vi "Page_Source_Can_Add_to_Top.vi"(6 "Project Refnum":refnum<vi>, 8 "error in (no error)":errorcluster, 10 "AB_Source in":refnum<class "AB_Source.lvclass">, 11 "AB_SourceDistribution in":refnum<class "AB_SourceDistribution.lvclass">) -> (0 "error out":errorcluster, 1 "message":string, 2 "canAddToTop":bool, 3 "AB_SourceDistribution out":refnum<class "AB_SourceDistribution.lvclass">)   [LabVIEW 2020, in "AB_SourceDistribution.lvclass"]
uses:
  <vilib>/AppBuilder/AB_Classes/SourceDistribution/AB_SourceDistribution.lvclass
  <vilib>/AppBuilder/AB_Classes/Source/AB_Source.lvclass
  <resource>/Framework/Providers/Common/provcom_StringGlobals.vi
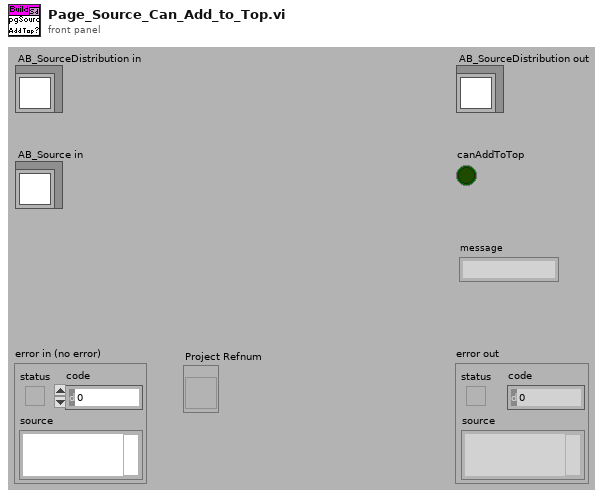
[diagram p1: front panel]
types:
  T1 = typedef "AB_Source.ctl" = cluster{"path":path, "itemID":string, "parentIndex":i32, "sourceInclusion":T2, "destinationIndex":i32, "properties":T3[], "newName":string, "lvfile":bool, "valid":bool, "eng_inBuild":bool, "eng_isNonVILink":bool, "Amalgamation":bool, "Amalgamation Piece":bool, "eng_delimitedName":string, "preventRename":bool}
  T2 = typedef "AB_Source_Inclusion.ctl" = enum16{"IncludeIfReferenced", "Include", "Exclude", "TopLevel"}
  T3 = typedef "AB_Source_Properties.ctl" = cluster{"sourcePropertyType":T4, "value":variant}
  T4 = typedef "AB_Source_Property_Type.ctl" = enum16{"Remove block diagram", "Remove front panel", "Password", "Window has title bar", "Show menu bar", "Show vertical scroll bar", "Show horizontal scroll bar", "Show toolbar", "Show Abort button", "Show fp when called", "Window behavior", "Allow user to close window", "Window run-time position", "Run when opened", "Allow debugging", "Auto error handling", "Generate guard code", "Use stack variables", "Expression folding", "Integer only", "Inline subVI"}
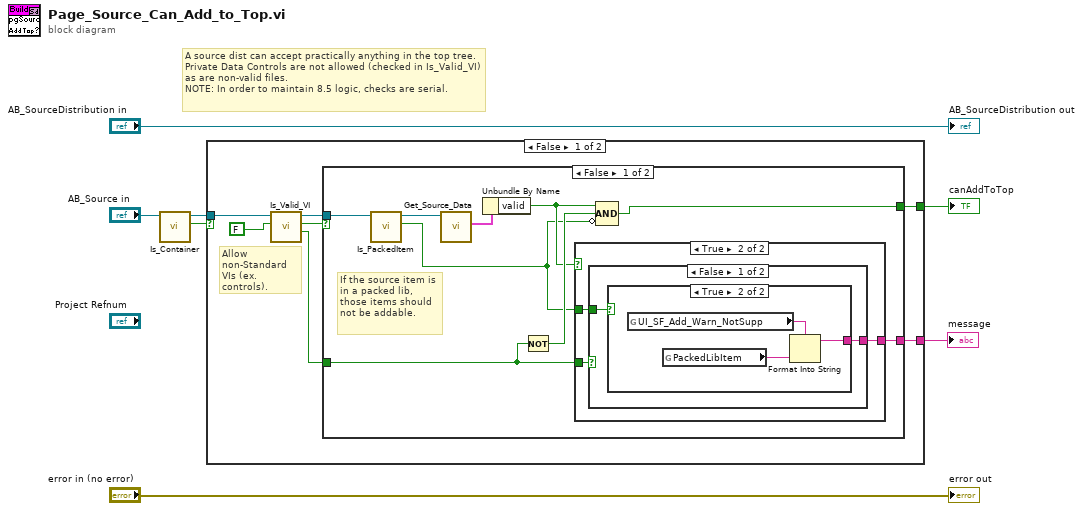
[diagram p0: block diagram]
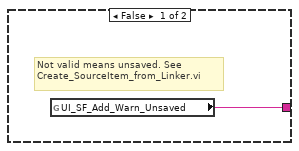
[diagram p2: hidden frame]
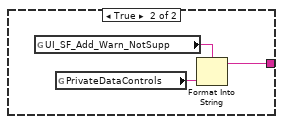
[diagram p4: hidden frame]
diagram:
  # "A source dist can accept practically anything in the top tree. Private Data Controls are not allowed (checked in Is_Valid_VI) as are non-valid files.\nNOTE: In order to maintain 8.5 logic, checks are serial."
  n1 = call-dynamic "Is_Container.vi"("AB_Source in"="AB_Source in") -> ("container"=w4:bool, "AB_Source out"=w2:refnum<class "AB_Source.lvclass">)  [unwired: 8 in, 1 out]
  n2 = case shown="False" w4 {
    selector: w4 -> [_ w37]
    tunnel: [w10 w37] -> w3
    tunnel: w2 -> [w14 _]
    tunnel: [w8 _] -> w1
    frame False {
      # "Allow non-Standard VIs (ex. controls)."
      n3 = call-dynamic "Is_Valid_VI.vi"("standardVI? (T)"=FALSE, "AB_Source in"=w14) -> ("PDC"=w9:bool, "VI"=w12:bool, "AB_Source out"=w11:refnum<class "AB_Source.lvclass">)  [unwired: 6 in, 1 out]
      n4 = case shown="False" w12 {
        selector: w12 -> [_ w36]
        tunnel: w11 -> [w17 _]
        tunnel: [w21 w36] -> w10
        tunnel: w9 -> [w18 _]
        tunnel: [w19 _] -> w8
        frame False {
          # "If the source item is in a packed lib, those items should not be addable."
          n5 = call-dynamic "Is_PackedItem.vi"("AB_Source in"=w17) -> ("packed item"=w15:bool, "AB_Source out"=w16:refnum<class "AB_Source.lvclass">)  [unwired: 8 in, 1 out]
          n6 = call <vilib>:"Get_Source_Data.vi"("Class in"=w16) -> ("data"=w23:T1)  [unwired: 8 in, 2 out]
          n7 = Unbundle By Name(w23) -> ("valid"=w20:bool)
          n8 = Not(x=w18) -> (.not. x?=w22:bool)
          n9 = case shown="True" w20 {
            tunnel: [w24 w26] -> w19
            tunnel: w18 -> [_ w27]
            tunnel: w15 -> [_ w25]
            frame False {
              # "Not valid means unsaved. See Create_SourceItem_from_Linker.vi"
              n10 = global read "provcom_StringGlobals.vi" "UI_SF_Add_Warn_Unsaved"() -> (w24:string)
            }
            frame True {
              n11 = case shown="False" w27 {
                tunnel: [w29 w33] -> w26
                tunnel: w25 -> [w28 _]
                frame False {
                  n12 = case shown="True" w28 {
                    tunnel: [_ w30] -> w29
                    frame False {
                      # "Should not hit this case."
                    }
                    frame True {
                      n13 = global read "provcom_StringGlobals.vi" "UI_SF_Add_Warn_NotSupp"() -> (w32:string)
                      n14 = global read "provcom_StringGlobals.vi" "PackedLibItem"() -> (w31:string)
                      n15 = Format Into String(format string=w32, w31) -> (resulting string=w30:string)  [unwired: 2 in, 1 out]
                    }
                  }
                }
                frame True {
                  n16 = global read "provcom_StringGlobals.vi" "UI_SF_Add_Warn_NotSupp"() -> (w35:string)
                  n17 = global read "provcom_StringGlobals.vi" "PrivateDataControls"() -> (w34:string)
                  n18 = Format Into String(format string=w35, w34) -> (resulting string=w33:string)  [unwired: 2 in, 1 out]
                }
              }
            }
          }
          n19 = Compound Arithmetic op=AND(w20, w22, invert w15) -> (w21:bool)
        }
        frame True {
        }
      }
    }
    frame True {
    }
  }
  "canAddToTop" <- w3
  "message" <- w1
  "error out" <- "error in (no error)"
  "AB_SourceDistribution out" <- "AB_SourceDistribution in"
